vi "VPA QC Assembly Checklist.vi"(10 "State Cluster":T1) -> (2 "State Cluster Out":T1)   [LabVIEW 2013]
uses:
  Controls/VPA QC State Data Cluster.ctl
  Controls/VPA QC General Cluster.ctl
  Controls/VPA QC State Enum.ctl
  Controls/VPA QC Bool Cluster.ctl
panel:
  in  "Done":bool
  in  "Voltage":bool caption="Ensure pump is running at the voltage specified by \ncustomer."
  in  "Wired":bool caption="Ensure that VPA is wired correctly."
  in  "Tighten Screws":bool
  in  "Drive Assem":bool caption="Ensure Drive Assembly checklist is complete."
  # "Drive Assembly Checklist"
  # "Assembly Checklist"
  # "Assembly Checklist"
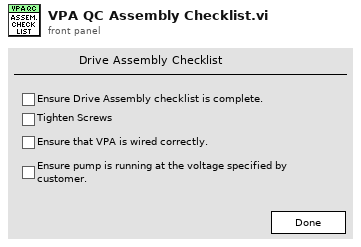
[diagram p1: front panel]
types:
  T1 = typedef "VPA QC State Data Cluster.ctl" = cluster{"XDCR 1":tag, "XDCR 2":tag, "General Information Clust":T2, "Assembly Checklist":cluster{"Ensure Drive Assembly checklist is completed.":bool, "Tighten Screws":bool, "Ensure VPA is wired correctly.":bool, "Ensure pump is running at voltage specified by customer.":bool}, "State":T3, "Manifold Leak Test Data":dbl[][], "Pressure Verification Test Data":dbl[][], "Flow Mode Verification Data":dbl[][], "DAQmx Error":errorcluster, "Bool Cluster":T4, "Leak Test Start Time":timestamp, "Pressure Test Start Time":timestamp, "Flow Test Start Time":timestamp, "Final Checklist cluster":cluster{"Check Fact Rest":bool, "Initialize Pump":bool, "Maintenance Hours":bool, "Clean Water Out":bool, "Covers":bool, "Screws":bool, "Wrap":bool, "Box":bool}, "Volts Constant":dbl, "Volume Constant A":dbl, "Volume Constant B":dbl, "Save File Path":path, "Comments Array":string[][], "File Format Version":u16}
  T2 = typedef "VPA QC General Cluster.ctl" = cluster{"Tech Name":string, "Date":timestamp, "Customer":string, "VPA Model":string, "G-72 Software Version":string, "Galil SN":string, "Galil Software Version":string, "VPA SN":string, "Valve SN":string, "Side A Drive Module SN":string, "Side B Drive Module SN":string, "A Side Transducer SN":string, "B Side Transducer SN":string, "A Side Motor SN":string, "B Side Motor SN":string, "A Side Gear Reducer SN":string, "B Side Gear Reducer SN":string, "A Side Limit Switch SN":string, "B Side Limit Switch SN":string, "Pump Voltage":string}
  T3 = typedef "VPA QC State Enum.ctl" = enum16{"General Information", "XDCR and LS Check", "Check Pump Function", "Manifold/Cylinder Leak Test", "Exit"}
  T4 = typedef "VPA QC Bool Cluster.ctl" = cluster{"Assembly":bool, "Gen":bool, "XDCR and LS Setup":bool, "Verify Pump Operation":bool, "Leak Test":bool, "Calibrate XDCRs":bool, "P Mode Verify":bool, "F Mode Verify":bool, "Vol Calibration":bool, "Flow Rate Test":bool, "Final Checklist":bool}
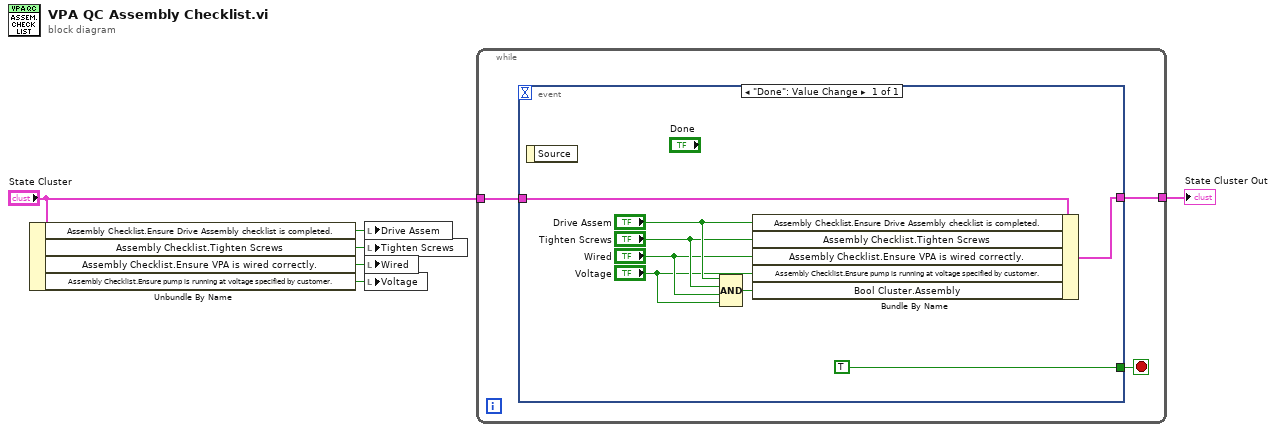
[diagram p0: block diagram]
diagram:
  n1 = Unbundle By Name("State Cluster") -> ("Assembly Checklist.Ensure Drive Assembly checklist is completed."=w2:bool, "Assembly Checklist.Tighten Screws"=w4:bool, "Assembly Checklist.Ensure VPA is wired correctly."=w3:bool, "Assembly Checklist.Ensure pump is running at voltage specified by customer."=w1:bool)
  n2 = local write "Drive Assem"(w2) -> ()
  n3 = local write "Tighten Screws"(w4) -> ()
  n4 = local write "Wired"(w3) -> ()
  n5 = local write "Voltage"(w1) -> ()
  n6 = while {
    tunnel: "State Cluster" -> [w8]
    tunnel: [w7] -> w6
    stop <- w9 stop-if-true
    n7 = event shown="[0] \"Done\": Value Change" {
      selector: _ -> [_]
      dyn-events: _ -> [_]
      timeout: _ -> [_]
      tunnel: [TRUE] -> w9
      tunnel: w8 -> [w16]
      tunnel: [w15] -> w7
      event "Done": Value Change {
        n8 = event-data() -> ()  [unwired: 1 in, 1 out]
        n9 = Compound Arithmetic op=AND("Drive Assem", "Tighten Screws", "Wired", "Voltage") -> (w10:bool)
        n10 = Bundle By Name(cluster=w16, "Assembly Checklist.Ensure Drive Assembly checklist is completed."="Drive Assem", "Assembly Checklist.Tighten Screws"="Tighten Screws", "Assembly Checklist.Ensure VPA is wired correctly."="Wired", "Assembly Checklist.Ensure pump is running at voltage specified by customer."="Voltage", "Bool Cluster.Assembly"=w10) -> (w15:T1)
      }
    }
  }
  "State Cluster Out" <- w6
